vi "ScannerMain.vi"() -> ()   [LabVIEW 2012]
uses:
  Strict Type Def - Scan Parameters Cluster.ctl
  Strict Type Def - Optimize Parameters Cluster.ctl
  Rabi Window Parameters.ctl
  ESR Window Parameters.ctl
  Spin Echo Window Parameters.ctl
  Window Parameters-CPMG.ctl
  SaveContrastOptions.ctl
  Window Parameters-XY4.ctl
  ESR Processing Params.ctl
  ESR Processing State.ctl
  ESR Modified Window Parameters.ctl
  States.ctl
  Global Vars.vi
  Channels.vi
panel:
  in  "Program":T1(tab)
  in  "Z Voltage":dbl min=-10.0 max=10.0 step=0.1
  in  "Continuous":bool
  in  "Green Laser (low-T)":bool caption="Scan"
  in  "Microwave":bool caption="Scan"
  in  "Green Laser":bool caption="Scan"
  out "Counts Intensity Graph":i32[][](graph)
  in  "Scan Parameters":T2={"X Max"=1.0, "X Min"=-1.0, "X Step"=0.01, "Y Max"=1.5, "Y Min"=-1.5, "Y Step"=0.015, "Dwell Time (ms) "=1} {"Dwell Time (ms)" min=0; "Y Step" min=0.0; "X Step" min=0.0}
  in  "Optimize":bool
  in  "Scan":bool
  in  "Count":bool caption="Optimize"
  out "Counts Chart":u32(graph)=76190
  out "Counts/s":i32=76190
  in  "Optimize Parameters":T3={"Volt Step"={"X"=0.005, "Y"=0.005, "Z"=0.01}, "Num Iterations"=5, "Dwell Time (ms)"=25, "Volts Range"={"X"=0.05, "Y"=0.05, "Z"=0.0}, "Method"={"X"=enum."Max", "Y"=enum."Max", "Z"=enum."Max"}} {"Volts Range"."Z" min=0.0; "Volts Range"."Y" min=0.0; "Volts Range"."X" min=0.0; "Dwell Time (ms)" min=0; "Num Iterations" min=1 step=1; "Volt Step"."Z" min=1e-05; "Volt Step"."Y" min=1e-06; "Volt Step"."X" min=1e-06}
  in  "ESR Post-Processing Parameters":T4={"Cut-off Threshhold"=1.3, "Processing Type"=enum."Off"}
  in  "ESR":bool caption="Scan"
  in  "ESR spectrum spreadsheet":path=path "C:/Users/Loncar/Dropbox/Raw data/2014-09-25 Measurements on R5C2L9 beam 9 NV/ESR_r5c2l9_beam9_55uW_m12dBm_oldPCBonSichips_hires.txt"
  in  "Save ESR spectrum data":bool
  in  "ESR spectrum graph":path=path "C:/Users/Loncar/Dropbox/Raw data/2014-09-25 Measurements on R5C2L9 beam 9 NV/ESR_r5c2l9_beam9_55uW_m12dBm_oldPCBonSichips_hires.jpg"
  in  "Save ESR spectrum graph":bool
  out "Avg ESR spectrum":cluster{"Y":dbl[], "Y":dbl[]}[](graph)=[{"Y"=[2.86, 2.8602499999999997, 2.8605, 2.86075, 2.8609999999999998, 2.86125, 2.8615, 2.86175, 2.862, 2.86225, 2.8625, 2.8627499999999997, 2.863, 2.86325, 2.8634999999999997, 2.86375, 2.864, 2.8642499999999997, 2.8645, 2.86475, 2.8649999999999998, 2.86525, 2.8655, 2.86575, 2.8659999999999997, 2.86625, 2.8665, 2.8667499999999997, 2.867, 2.86725, 2.8674999999999997, 2.86775, 2.868, 2.8682499999999997, 2.8685, 2.86875, 2.8689999999999998, 2.86925, 2.8695, 2.86975, 2.87, 2.87025, 2.8705, 2.8707499999999997, 2.871, 2.87125, 2.8714999999999997, 2.87175, 2.872, 2.8722499999999997, 2.8725, 2.87275, 2.8729999999999998, 2.87325, 2.8735, 2.87375, 2.8739999999999997, 2.87425, 2.8745, 2.8747499999999997, 2.875, 2.87525, 2.8754999999999997, 2.87575, 2.876, 2.8762499999999998, 2.8765, 2.87675, 2.877, 2.87725, 2.8775, 2.87775, 2.878, 2.87825, 2.8785, 2.8787499999999997, 2.879, 2.87925, 2.8794999999999997, 2.87975, 2.88], "Y"=[171.2, 172.675, 175.59166666666667, 174.09166666666667, 175.0, 174.94166666666666, 175.05833333333334, 176.20833333333334, 174.75833333333333, 172.9, 173.675, 175.35, 174.325, 172.54166666666666, 173.83333333333334, 172.03333333333333, 173.89166666666668, 174.84166666666667, 173.04166666666666, 173.16666666666666, 171.03333333333333, 171.68333333333334, 169.74166666666667, 168.125, 167.25833333333333, 165.89166666666668, 163.9, 160.34166666666667, 155.55, 154.05, 152.5, 153.3, 153.525, 157.55833333333334, 161.56666666666666, 157.38333333333333, 157.175, 158.2, 154.24166666666667, 152.09166666666667, 147.9, 147.6, 147.875, 147.125, 149.8, 152.39166666666668, 156.35, 154.675, 157.55833333333334, 161.69166666666666, 160.13333333333333, 160.275, 160.2, 156.75833333333333, 156.76666666666668, 152.64166666666668, 149.14166666666668, 153.64166666666668, 155.76666666666668, 158.53333333333333, 162.56666666666666, 165.725, 168.45, 166.98333333333332, 168.93333333333334, 171.05833333333334, 172.13333333333333, 171.3, 172.825, 172.78333333333333, 171.06666666666666, 173.50833333333333, 171.28333333333333, 173.075, 172.475, 171.44166666666666, 173.40833333333333, 175.19166666666666, 172.86666666666667, 174.90833333333333, 174.175]}]
  out "Counts vs. frequency":i32[][](graph)
  in  "# freq points":i32=81
  in  "MW start freq (GHz)":dbl=2.86
  in  "MW stop freq (GHz)":dbl=2.88
  in  "# scans before track":i32=20
  in  "#scan iterations":i32=20
  in  "ESR Parameters":T6={"Window 1 time (s)"=0.012, "Window 2 time (s)"=5e-06, "Window 3 time (s) "=0.02, "Window 4 time (s)"=5e-07, "Window 4 channels"=[FALSE, FALSE, FALSE, TRUE], "Window 3 channels"=[FALSE, FALSE, TRUE, TRUE], "Window 2 channels"=[FALSE, FALSE, FALSE, TRUE], "Window 1 channels"=[FALSE, TRUE, FALSE, TRUE], "Path to ESR Burner"=path "C:/Users/Loncar/Desktop/ESR VIs - Srujan/Sam Kim/PB/ESRFreq.exe"}
  in  "ESR Save Data 2":T7={"Save avg spectrum graph"=FALSE, "Path for avg spectrum graph"=path "C:/experiment/data/may_15_2012/SIL1_NV1_pippin_uW_off", "Save data to spreadsheet"=FALSE, "Path for avg spectrum spreadsheet"=path "C:/experiment/data/may_15_2012/SIL1_NV1_pippin_uW_off"}
  out "Avg ESR spectrum 2-2":cluster{"Y":dbl[], "Y":dbl[]}[](graph)=[{"Y"=[2.86, 2.8602499999999997, 2.8605, 2.86075, 2.8609999999999998, 2.86125, 2.8615, 2.86175, 2.862, 2.86225, 2.8625, 2.8627499999999997, 2.863, 2.86325, 2.8634999999999997, 2.86375, 2.864, 2.8642499999999997, 2.8645, 2.86475, 2.8649999999999998, 2.86525, 2.8655, 2.86575, 2.8659999999999997, 2.86625, 2.8665, 2.8667499999999997, 2.867, 2.86725, 2.8674999999999997, 2.86775, 2.868, 2.8682499999999997, 2.8685, 2.86875, 2.8689999999999998, 2.86925, 2.8695, 2.86975, 2.87, 2.87025, 2.8705, 2.8707499999999997, 2.871, 2.87125, 2.8714999999999997, 2.87175, 2.872, 2.8722499999999997, 2.8725, 2.87275, 2.8729999999999998, 2.87325, 2.8735, 2.87375, 2.8739999999999997, 2.87425, 2.8745, 2.8747499999999997, 2.875, 2.87525, 2.8754999999999997, 2.87575, 2.876, 2.8762499999999998, 2.8765, 2.87675, 2.877, 2.87725, 2.8775, 2.87775, 2.878, 2.87825, 2.8785, 2.8787499999999997, 2.879, 2.87925, 2.8794999999999997, 2.87975, 2.88], "Y"=[171.2, 172.675, 175.59166666666667, 174.09166666666667, 175.0, 174.94166666666666, 175.05833333333334, 176.20833333333334, 174.75833333333333, 172.9, 173.675, 175.35, 174.325, 172.54166666666666, 173.83333333333334, 172.03333333333333, 173.89166666666668, 174.84166666666667, 173.04166666666666, 173.16666666666666, 171.03333333333333, 171.68333333333334, 169.74166666666667, 168.125, 167.25833333333333, 165.89166666666668, 163.9, 160.34166666666667, 155.55, 154.05, 152.5, 153.3, 153.525, 157.55833333333334, 161.56666666666666, 157.38333333333333, 157.175, 158.2, 154.24166666666667, 152.09166666666667, 147.9, 147.6, 147.875, 147.125, 149.8, 152.39166666666668, 156.35, 154.675, 157.55833333333334, 161.69166666666666, 160.13333333333333, 160.275, 160.2, 156.75833333333333, 156.76666666666668, 152.64166666666668, 149.14166666666668, 153.64166666666668, 155.76666666666668, 158.53333333333333, 162.56666666666666, 165.725, 168.45, 166.98333333333332, 168.93333333333334, 171.05833333333334, 172.13333333333333, 171.3, 172.825, 172.78333333333333, 171.06666666666666, 173.50833333333333, 171.28333333333333, 173.075, 172.475, 171.44166666666666, 173.40833333333333, 175.19166666666666, 172.86666666666667, 174.90833333333333, 174.175]}] caption="Avg ESR spectrum 2"
  out "Counts vs. frequency 2-2":i32[][](graph) caption="Counts vs. frequency 2"
  in  "ESR Save Data 1":T7={"Save avg spectrum graph"=FALSE, "Path for avg spectrum graph"=path "C:/experiment/data/may_15_2012/SIL1_NV1_pippin_uW_off", "Save data to spreadsheet"=FALSE, "Path for avg spectrum spreadsheet"=path "C:/experiment/data/may_15_2012/SIL1_NV1_pippin_uW_off"}
  in  "ESR Post-Processing Parameters 2":T4={"Cut-off Threshhold"=1.3, "Processing Type"=enum."Off"}
  in  "ESR 2":bool caption="Scan"
  out "Avg ESR spectrum 2-1":cluster{"Y":dbl[], "Y":dbl[]}[](graph)=[{"Y"=[2.86, 2.8602499999999997, 2.8605, 2.86075, 2.8609999999999998, 2.86125, 2.8615, 2.86175, 2.862, 2.86225, 2.8625, 2.8627499999999997, 2.863, 2.86325, 2.8634999999999997, 2.86375, 2.864, 2.8642499999999997, 2.8645, 2.86475, 2.8649999999999998, 2.86525, 2.8655, 2.86575, 2.8659999999999997, 2.86625, 2.8665, 2.8667499999999997, 2.867, 2.86725, 2.8674999999999997, 2.86775, 2.868, 2.8682499999999997, 2.8685, 2.86875, 2.8689999999999998, 2.86925, 2.8695, 2.86975, 2.87, 2.87025, 2.8705, 2.8707499999999997, 2.871, 2.87125, 2.8714999999999997, 2.87175, 2.872, 2.8722499999999997, 2.8725, 2.87275, 2.8729999999999998, 2.87325, 2.8735, 2.87375, 2.8739999999999997, 2.87425, 2.8745, 2.8747499999999997, 2.875, 2.87525, 2.8754999999999997, 2.87575, 2.876, 2.8762499999999998, 2.8765, 2.87675, 2.877, 2.87725, 2.8775, 2.87775, 2.878, 2.87825, 2.8785, 2.8787499999999997, 2.879, 2.87925, 2.8794999999999997, 2.87975, 2.88], "Y"=[171.2, 172.675, 175.59166666666667, 174.09166666666667, 175.0, 174.94166666666666, 175.05833333333334, 176.20833333333334, 174.75833333333333, 172.9, 173.675, 175.35, 174.325, 172.54166666666666, 173.83333333333334, 172.03333333333333, 173.89166666666668, 174.84166666666667, 173.04166666666666, 173.16666666666666, 171.03333333333333, 171.68333333333334, 169.74166666666667, 168.125, 167.25833333333333, 165.89166666666668, 163.9, 160.34166666666667, 155.55, 154.05, 152.5, 153.3, 153.525, 157.55833333333334, 161.56666666666666, 157.38333333333333, 157.175, 158.2, 154.24166666666667, 152.09166666666667, 147.9, 147.6, 147.875, 147.125, 149.8, 152.39166666666668, 156.35, 154.675, 157.55833333333334, 161.69166666666666, 160.13333333333333, 160.275, 160.2, 156.75833333333333, 156.76666666666668, 152.64166666666668, 149.14166666666668, 153.64166666666668, 155.76666666666668, 158.53333333333333, 162.56666666666666, 165.725, 168.45, 166.98333333333332, 168.93333333333334, 171.05833333333334, 172.13333333333333, 171.3, 172.825, 172.78333333333333, 171.06666666666666, 173.50833333333333, 171.28333333333333, 173.075, 172.475, 171.44166666666666, 173.40833333333333, 175.19166666666666, 172.86666666666667, 174.90833333333333, 174.175]}] caption="Avg ESR spectrum 1"
  out "Counts vs. frequency 2-1":i32[][](graph) caption="Counts vs. frequency 1"
  in  "# freq points 2":i32=81 caption="# freq points"
  in  "MW start freq (GHz) 2":dbl=2.86 caption="MW start freq (GHz)"
  in  "MW stop freq (GHz) 2":dbl=2.88 caption="MW stop freq (GHz)"
  in  "# scans before track 2":i32=20
  in  "#scan iterations 2":i32=20 caption="#scan iterations"
  in  "ESR Modified Parameters":T8={"Window 1 time (s)"=0.012, "Window 2 time (s)"=5e-06, "Window 3 time (s) "=0.02, "Window 4 time (s)"=5e-07, "Window 4 channels"=[FALSE, FALSE, FALSE, TRUE], "Window 3 channels"=[FALSE, FALSE, TRUE, TRUE], "Window 2 channels"=[FALSE, FALSE, FALSE, TRUE], "Window 1 channels"=[FALSE, TRUE, FALSE, TRUE], "Path to ESR Burner"=path "C:/Users/Loncar/Desktop/ESR VIs - Srujan/Sam Kim/PB/ESR_modified_burn.exe", "Window 5 time (s)"=1.0, "Drive channel"=4} {"Drive channel" max=8}
  out "Rabi # scans done":u32=4
  in  "Save Rabi Contrast Options":T9={"Save contrast graph"=FALSE, "Path for contrast graph"=path "C:/Users/Loncar/Dropbox/Raw data/2014-09-25 Measurements on R5C2L9 beam 9 NV/Rabi_r5c2l9_beam9_100uW_3dBm2p87050GHz_oldPCBonSichips.jpg", "Save contrast data"=FALSE, "Path for contrast data"=path "C:/Users/Loncar/Dropbox/Raw data/2014-09-25 Measurements on R5C2L9 beam 9 NV/Rabi_r5c2l9_beam9_100uW_3dBm2p87050GHz_oldPCBonSichips.txt"}
  in  "# scan iterations":i32=100
  in  "Rabi Parameters":T10={"Window 1 time (s)"=3e-06, "Window 2 time (s)"=1e-06, "Window 3 min time (s) "=1.2e-08, "Window 3 max time (s)"=2e-07, "Window 4 time (s)"=7.5e-07, "Window 5 time (s)"=2e-07, "Window 6 time (s)"=3e-06, "Window 7 time (s)"=2e-07, "Window 8 time (s)"=1e-07, "# samples before track"=100000, "# time axis points"=94, "Window 1 active channels"=[TRUE, FALSE, FALSE, TRUE], "Window 2 active channels"=[TRUE], "Window 3 active channels"=[FALSE], "Window 4 active channels"=[TRUE, FALSE, FALSE, TRUE], "Window 5 active channels "=[TRUE, FALSE, TRUE, TRUE], "Window 6 active channels"=[TRUE, FALSE, FALSE, TRUE], "Window 7 active channels"=[TRUE, FALSE, TRUE, TRUE], "Window 8 active channels"=[TRUE], "Path to Rabi Burner"=path "C:/Users/Loncar/Desktop/ESR VIs - Srujan/Sam Kim/PB/RabiBurn.exe"}
  out "Rabi Normalized contrast":cluster{"Y":dbl[], "Y":dbl[]}[](graph)=[{"Y"=[0.012, 0.014021505376344086, 0.016043010752688172, 0.018064516129032256, 0.020086021505376344, 0.02210752688172043, 0.024129032258064516, 0.0261505376344086, 0.028172043010752684, 0.030193548387096772, 0.03221505376344086, 0.03423655913978495, 0.03625806451612903, 0.038279569892473116, 0.0403010752688172, 0.04232258064516129, 0.04434408602150538, 0.04636559139784946, 0.04838709677419355, 0.050408602150537635, 0.05243010752688172, 0.05445161290322581, 0.05647311827956989, 0.05849462365591398, 0.06051612903225806, 0.06253763440860215, 0.06455913978494623, 0.06658064516129032, 0.0686021505376344, 0.0706236559139785, 0.07264516129032259, 0.07466666666666666, 0.07668817204301075, 0.07870967741935485, 0.08073118279569892, 0.08275268817204301, 0.0847741935483871, 0.08679569892473118, 0.08881720430107527, 0.09083870967741935, 0.09286021505376345, 0.09488172043010752, 0.09690322580645161, 0.0989247311827957, 0.10094623655913978, 0.10296774193548387, 0.10498924731182795, 0.10701075268817205, 0.10903225806451612, 0.11105376344086021, 0.1130752688172043, 0.11509677419354838, 0.11711827956989247, 0.11913978494623655, 0.12116129032258065, 0.12318279569892474, 0.1252043010752688, 0.12722580645161288, 0.12924731182795698, 0.13126881720430106, 0.13329032258064516, 0.13531182795698926, 0.1373333333333333, 0.1393548387096774, 0.1413763440860215, 0.14339784946236558, 0.14541935483870969, 0.14744086021505376, 0.14946236559139783, 0.15148387096774193, 0.15350537634408604, 0.1555268817204301, 0.15754838709677418, 0.15956989247311826, 0.16159139784946236, 0.16361290322580646, 0.16563440860215053, 0.1676559139784946, 0.1696774193548387, 0.17169892473118278, 0.17372043010752689, 0.175741935483871, 0.17776344086021503, 0.17978494623655913, 0.1818064516129032, 0.1838279569892473, 0.1858494623655914, 0.18787096774193546, 0.18989247311827956, 0.19191397849462366, 0.19393548387096773, 0.19595698924731184, 0.1979784946236559, 0.19999999999999998], "Y"=[-0.08553971486761709, 0.011664899257688167, 0.13925438596491221, 0.06770255271920085, 0.08048511576626233, -0.04601226993865021, 0.030916844349680114, -0.032734952481520585, 0.02651933701657463, 0.013978494623655904, -0.07476635514018694, 0.012074643249176665, 0.015856236786469385, -0.016685205784204595, -0.03520352035203522, -0.0965447154471545, -0.10626992561105213, -0.11300639658848623, -0.09570957095709565, -0.12087912087912084, -0.17196056955093092, -0.12861736334405144, -0.1610169491525424, -0.12705366922234393, -0.10515463917525783, -0.1439312567132116, -0.09857612267250825, -0.08786127167630059, -0.14553472987872113, -0.1956521739130434, -0.19296375266524526, -0.23037716615698273, -0.23809523809523814, -0.2172489082969433, -0.25467775467775466, -0.22137404580152667, -0.30620985010706636, -0.23583934088568478, -0.30512016718913265, -0.31137088204038255, -0.2988260405549626, -0.21221864951768493, -0.2749731471535982, -0.29181084198385243, -0.31327800829875513, -0.3020719738276989, -0.20136518771331055, -0.38453713123092575, -0.3240641711229947, -0.3050483351235231, -0.41277890466531436, -0.37362637362637363, -0.3563096500530223, -0.3563714902807775, -0.3038793103448276, -0.3427922814982974, -0.39764201500535906, -0.3432203389830508, -0.37060702875399354, -0.2960893854748603, -0.3371017471736897, -0.3094462540716613, -0.3705636743215031, -0.37731958762886597, -0.3152866242038217, -0.2636871508379888, -0.35586481113320073, -0.29205366357069146, -0.34840698869475845, -0.35966735966735963, -0.36185567010309283, -0.2676537585421412, -0.3159541188738269, -0.30687830687830686, -0.3009605122732124, -0.29538131041890436, -0.24860646599777034, -0.2631578947368421, -0.26400862068965514, -0.3076923076923076, -0.208955223880597, -0.2309322033898305, -0.29610115911485774, -0.23751274209989817, -0.20000000000000007, -0.18343815513626838, -0.23179487179487177, -0.2694248234106962, -0.1670258620689655, -0.2071503680336488, -0.20141700404858295, -0.17057569296375263, -0.1054384017758047, -0.15129533678756485]}]
  in  "Rabi":bool caption="Scan"
  in  "Rabi Pause":bool
  out "Rabi Last counts/s":u32 caption="Last counts/s"
  out "Last counts/s":u32
  out "SpinEcho scans done":u32=104
  in  "Pause Spin Echo":bool
  in  "SpinEcho Save Options":T9={"Save contrast graph"=FALSE, "Path for contrast graph"=path "C:/Users/Loncar/Dropbox/Raw data/2014-09-25 Measurements on R5C2L9 beam 9 NV/SpinEcho_r5c2l9_beam9_100uW_3dBm2p87050GHz_oldPCBonSichips_10us.jpg", "Save contrast data"=FALSE, "Path for contrast data"=path "C:/Users/Loncar/Dropbox/Raw data/2014-09-25 Measurements on R5C2L9 beam 9 NV/SpinEcho_r5c2l9_beam9_100uW_3dBm2p87050GHz_oldPCBonSichips_10us.txt"}
  in  "# SpinEcho scan iterations":i32=200
  in  "Spin Echo Parameters":T11={"Path to Spin Echo Burner"=path "C:/Users/Loncar/Desktop/ESR VIs - Srujan/Sam Kim/PB/SpinEchoBurn.exe", "Window 1 time (s)"=3e-06, "Window 1 active channels"=[TRUE, FALSE, FALSE, TRUE], "Window 10 time (s)"=3e-06, "Window 10 active channels"=[TRUE, FALSE, FALSE, TRUE], "# samples"=50000, "Window 2 time (s)"=1e-06, "Window 2 active channels"=[TRUE], "Window 4 min time (s) "=1.2e-08, "Window 4 active channels"=[TRUE], "Window 8 time (s)"=7.5e-07, "Window 8 active channels"=[TRUE, FALSE, FALSE, TRUE], "Window 9 time (s)"=2e-07, "Window 9 active channels "=[TRUE, FALSE, TRUE, TRUE], "# time axis points"=300, "Window 11 time (s)"=2e-07, "Window 11 active channels"=[TRUE, FALSE, TRUE, TRUE], "Window 12 time (s)"=1e-07, "Window 12 active channels"=[TRUE], "Window 4 max time (s)"=1e-05, "Window 3 time (s)"=6.5e-08, "Window 5 time (s)"=2.6e-07, "Window 3 active channels"=[FALSE, FALSE, FALSE, FALSE], "Window 5 active channels"=[FALSE, FALSE, FALSE, FALSE], "Window 7 time (s)"=6.5e-08, "Window 7 active channels"=[FALSE, FALSE, FALSE, FALSE]}
  out "Spin Echo contrast":cluster{"Y":dbl[], "Y":dbl[]}[](graph)
  in  "Spin Echo":bool caption="Scan"
  out "CPMG scans done":u32=88
  in  "Save CPMG Contrast Options":T9={"Save contrast graph"=FALSE, "Path for contrast graph"=path "C:/Users/Public/Documents/Srujan/2014-06-22/NV3_CPMG_n2_2p83GHz3dBm_pi64ns_100us.jpg", "Save contrast data"=FALSE, "Path for contrast data"=path "C:/Users/Public/Documents/Srujan/2014-06-22/NV3_CPMG_n2_2p83GHz3dBm_pi64ns_100us.txt"}
  out "CPMG contrast":cluster{"Y":dbl[], "Y":dbl[]}[](graph)
  in  "CPMG":bool caption="Scan"
  in  "# scan iterations":i32=200
  in  "CPMG Parameters":T12={"Path to CPMG Burner"=path "C:/Users/Loncar/Desktop/ESR VIs - Srujan/Sam Kim/PB/SpinEchoBurn.exe", "Window 1 time (s)"=3e-06, "Window 1 active channels"=[FALSE, FALSE, FALSE, TRUE], "Window 10 time (s)"=3e-06, "Window 10 active channels"=[FALSE, FALSE, FALSE, TRUE], "Window 2 time (s)"=1e-06, "Window 2 active channels"=[], "Window 4 min time (s) "=1.2e-08, "Window 4 active channels"=[FALSE], "Window 8 time (s)"=7.5e-07, "Window 8 active channels"=[FALSE, FALSE, FALSE, TRUE], "Window 9 time (s)"=3e-07, "Window 9 active channels "=[FALSE, FALSE, TRUE, TRUE], "# delay time points"=100, "Window 11 time (s)"=3e-07, "Window 11 active channels"=[FALSE, FALSE, TRUE, TRUE], "Window 12 time (s)"=1e-07, "Window 12 active channels"=[], "Window 4 max time (s)"=0.0001, "Window 3 time (s)"=3.2e-08, "Window 5 time (s)"=6.4e-08, "Window 3 active channels"=[TRUE, FALSE, FALSE, FALSE], "Window 5 active channels"=[TRUE, FALSE, FALSE, FALSE], "# pi pulses"=2, "# samples before track"=20000} {"# pi pulses" min=1; "# delay time points" min=2}
  in  "Save XY-4 Contrast Options":T9={"Save contrast graph"=FALSE, "Path for contrast graph"=path "C:/experiment/data/may_15_2012/SIL1_NV1_pippin_uW_off", "Save contrast data"=FALSE, "Path for contrast data"=path "C:/experiment/data/may_15_2012/SIL1_NV1_pippin_uW_off"}
  out "XY-4 Normalized contrast":cluster{"Y":dbl[], "Y":dbl[]}[](graph)
  in  "XY-4":bool caption="Scan"
  in  "# scan iterations":i32
  in  "XY-4 Parameters":T13={"Path to CPMG Burner"=path "C:/Users/Loncar/Desktop/ESR VIs - Srujan/Sam Kim/PB/SpinEchoBurn.exe", "Window 1 time (s)"=3e-06, "Window 1 active channels"=[FALSE, FALSE, FALSE, TRUE], "Window 10 time (s)"=3e-06, "Window 10 active channels"=[FALSE, FALSE, FALSE, TRUE], "Window 2 time (s)"=0.0, "Window 2 active channels"=[], "Window 4 min time (s) "=0.0, "Window 4 active channels"=[FALSE], "Window 8 time (s)"=7.5e-07, "Window 8 active channels"=[FALSE, FALSE, FALSE, TRUE], "Window 9 time (s)"=2e-07, "Window 9 active channels "=[FALSE, FALSE, TRUE, TRUE], "# time points"=2, "Window 11 time (s)"=0.0, "Window 11 active channels"=[FALSE, FALSE, TRUE, TRUE], "Window 12 time (s)"=1e-07, "Window 12 active channels"=[], "Window 4 max time (s)"=0.0, "Window 3 time (s)"=0.0, "Window 5 time (s)"=5e-06, "Window 3 active channels"=[TRUE, FALSE, FALSE, FALSE], "Window 5c active channels"=[TRUE, FALSE, FALSE, FALSE], "# pulse sequences"=1, "# samples before track"=0, "Window 5a active channels"=[TRUE, FALSE, FALSE, FALSE]} {"# pulse sequences" min=1; "# time points" min=2}
  in  "Z AO Channel":tag="Dev1/ao2"
  in  "Laser voltage":tag="Dev1/ao2"
  in  "Counter(s)":tag="Dev1/ctr0"
  in  "X AO Channel":tag="Dev1/ao0"
  in  "Y AO Channel":tag="Dev1/ao1"
  in  "Sample clock line":tag="/Dev1/PFI9"
  in  "spinapi.dll":path=path "C:/SpinCore/SpinAPI/dll/spinapi64.dll"
  in  "HoldChannel.exe":path=path "C:/Users/Loncar/Desktop/ESR VIs - Srujan/Sam Kim/PB/HoldChannel.exe"
  # "Note for Z: 1 V = 10 um"
  # "X, Y, and Z display values\nonly update after manual\noptimization"
  # "Default PB connections:\nPB0 - MW switch\nPB3 - Green AOM\n\nDefault for low-T:\nPB1 - Green AOM"
  # "ESR spectrum measurement"
  # "Default PB connections:\nPB0 - MW switch\nPB1 - MW freq step\nPB2 - Counter sample clk\nPB3 - Green AOM"
  # "Pulse sequence parameters - Window durations and PB channel states"
  # "Green AOM, MW switch are always on!"
  # "(to spreadsheet)"
  # "Remove Outlier Scan: If there are outlier data\n    in a scan, then removes that scan\nRemove Outlier Data: If there are outlier data,\n    then replaces the data with the mean of\n    that scan"
  # "* <data>"
  # "MW freq step\ndwell time"
  # "MW freq step"
  # "Wait"
  # "Fluorescence\ncounting"
  # "Ctr sample clk"
  # "Wait"
  # "ESR 2 (modified) measurement"
  # "Default PB connections:\nPB0 - MW switch\nPB1 - MW freq step\nPB2 - Counter sample clk\nPB3 - Green AOM\nPB4 - Piezo drive"
  # "Modified version: Alternates frequency sweep with channel on/off for driving cantilever"
  # "Pulse sequence parameters - Window durations and PB channel states"
  # "Green AOM, MW switch are always on!"
  # "Remove Outlier Scan: If there are outlier data\n    in a scan, then removes that scan\nRemove Outlier Data: If there are outlier data,\n    then replaces the data with the mean of\n    that scan"
  # "* <data>"
  # "MW freq step\ndwell time"
  # "MW freq step"
  # "Wait"
  # "Fluorescence\ncounting"
  # "Ctr sample clk"
  # "Wait"
  # "Wait between\nfreq sweeps"
  # "On/off between freq sweeps (off first)"
  # "Rabi measurement"
  # "Default PB connections:\nPB0 - MW switch\nPB1 - unused\nPB2 - Counter sample clk\nPB3 - Green AOM"
  # "to spreadsheet"
  # "Initialization"
  # "Green AOM"
  # "Wait"
  # "All off"
  # "MW pulsing"
  # "MW"
  # "Wait"
  # "Green AOM"
  # "Green AOM,\ncounter clk"
  # "Readout"
  # "Repump"
  # "Green AOM"
  # "Green AOM,\ncounter clk"
  # "Reference"
  # "All off"
  # "Wait (nominal)"
  # "Spin Echo measurement"
  # "Default PB connections:\nPB0 - MW switch\nPB1 - unused\nPB2 - Counter sample clk\nPB3 - Green AOM"
  # "to spreadsheet"
  # "Green AOM"
  # "Initialization"
  # "All off"
  # "Wait"
  # "MW"
  # "MW pulse 1"
  # "All off"
  # "Free precession 1"
  # "max: ~350"
  # "MW pulse 2"
  # "MW"
  # "Free precession 2: Window 6"
  # "MW"
  # "MW pulse 1"
  # "Green AOM"
  # "Wait"
  # "Green AOM,\ncounter clk"
  # "Readout"
  # "Green AOM"
  # "Repump"
  # "Green AOM,\ncounter clk"
  # "Reference"
  # "Wait (nominal)"
  # "All off"
  # "CPMG measurement"
  # "Default PB connections:\nPB0 - MW switch\nPB1 - MW 90deg phase shifted\nPB2 - Counter sample clk\nPB3 - Green AOM"
  # "to spreadsheet"
  # "Green AOM"
  # "Initialization"
  # "All off"
  # "Wait"
  # "MW pulse 1\n(pi/2)"
  # "MW"
  # "Free precession\n(Tau/2)"
  # "All off"
  # "max: ~350"
  # "MW pulse 2\n(pi90)"
  # "MW90"
  # "Free precession (Tau/2)\nMW pulse 1 (pi/2)"
  # "Window 6 = Window 4\nWindow 7 = Window 3"
  # "All off\nMW"
  # "Green AOM"
  # "Wait for green"
  # "Green AOM,\ncounter clk"
  # "Readout"
  # "Green AOM"
  # "Repump"
  # "Green AOM,\ncounter clk"
  # "Reference"
  # "Wait (nominal)"
  # "All off"
  # "XY-4 measurement"
  # "Default PB connections:\nPB0 - MW switch\nPB1 - MW 90deg phase shifted\nPB2 - Counter sample clk\nPB3 - Green AOM"
  # "to spreadsheet"
  # "pulse=XYXY"
  # "max: ~350"
  # "x 4=#pi pulses"
  # "Green AOM"
  # "Initialization"
  # "All off"
  # "Wait"
  # "MW pulse 1\n(pi/2)"
  # "MW"
  # "Free precession\n(T/2)"
  # "All off"
  # "MW (X)"
  # "MW pulse 2\n(pi)"
  # "MW90 (Y)"
  # "Pulse Sequence=[T/2-Pi-T-Pi90-T-Pi-T-Pi90-T/2]^N\nMW pulse 1 (pi/2)"
  # "Window 4-5a-g-6\nWindow 7"
  # "Green AOM"
  # "Wait for green"
  # "Green AOM,\ncounter sample clk"
  # "Readout"
  # "Green AOM"
  # "Repump"
  # "Green AOM,\ncounter sample clk"
  # "Reference"
  # "Wait (nominal)"
  # "All off"
  # "TODO:\nHigh priority:\n(done) Show counts during pulsed experiments\nFigure out off-by-1 error in raster scan(?)\nImplement scanning with second arm\n\nMedium priority:\nChanges in Srujan's low-T experiments\n\nLow priority:\nContinuous Scan does not save image\nSave Counts Intensity Graph as image to clipbard\nAllow ESR+pulsed experiments to stop and save\n    (1. Stop at end of run; 2. Force stop)\nImplement new tracking algorithm for noisy data\n    (Ensemble NV centers)\nAllow stopping in middle of optimize\nAllow count concurrently with optimize/scan(?)"
  # "Author: Samuel Kim\nESR, Rabi, and Spin Echo experiments adapted from Srujan"
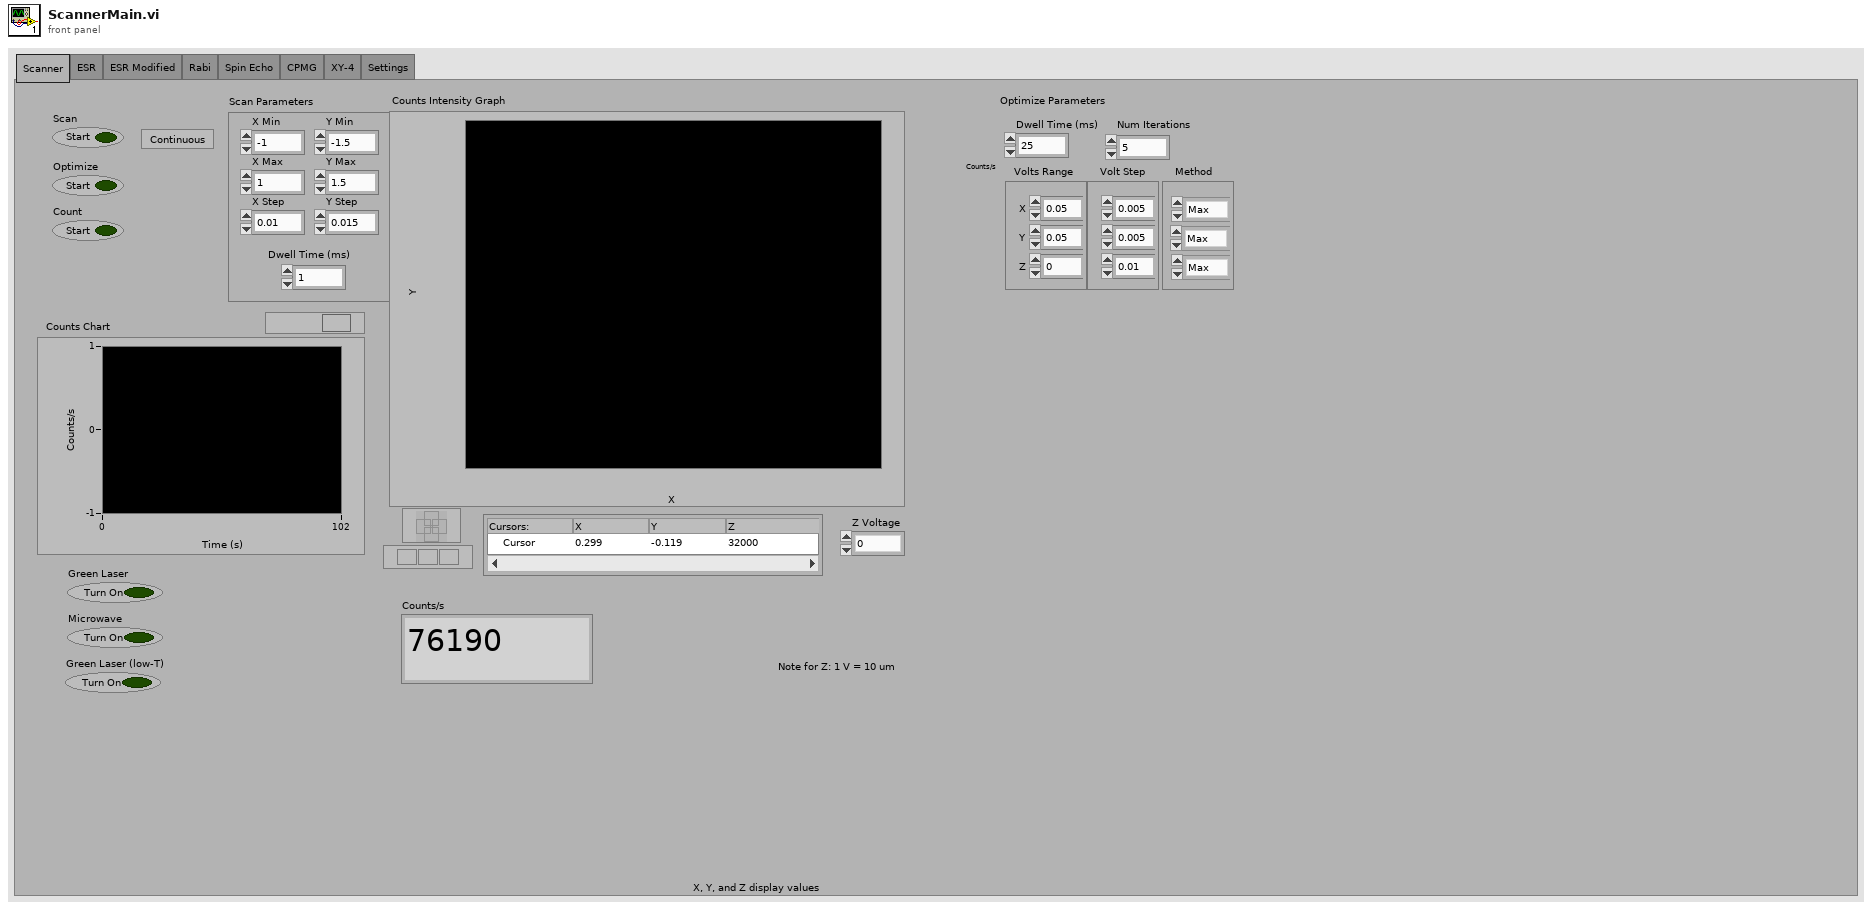
[diagram p1: front panel]
types:
  T1 = enum32{"Scanner", "ESR", "ESR Modified", "Rabi", "Spin Echo", "CPMG", "XY-4", "Settings"}
  T2 = typedef "Strict Type Def - Scan Parameters Cluster.ctl" = cluster{"X Max":dbl, "X Min":dbl, "X Step":dbl, "Y Max":dbl, "Y Min":dbl, "Y Step":dbl, "Dwell Time (ms) ":i32}
  T3 = typedef "Strict Type Def - Optimize Parameters Cluster.ctl" = cluster{"Volt Step":cluster{"X":dbl, "Y":dbl, "Z":dbl}, "Num Iterations":i32, "Dwell Time (ms)":i32, "Volts Range":cluster{"X":dbl, "Y":dbl, "Z":dbl}, "Method":cluster{"X":enum16{"Max", "Gaussian"}, "Y":enum16{"Max", "Gaussian"}, "Z":enum16{"Max", "Gaussian"}}}
  T4 = typedef "ESR Processing Params.ctl" = cluster{"Cut-off Threshhold":dbl, "Processing Type":T5}
  T5 = typedef "ESR Processing State.ctl" = enum16{"Off", "Remove Outlier Scan", "Remove Outlier Data"}
  T6 = typedef "ESR Window Parameters.ctl" = cluster{"Window 1 time (s)":dbl, "Window 2 time (s)":dbl, "Window 3 time (s) ":dbl, "Window 4 time (s)":dbl, "Window 4 channels":bool[], "Window 3 channels":bool[], "Window 2 channels":bool[], "Window 1 channels":bool[], "Path to ESR Burner":path}
  T7 = cluster{"Save avg spectrum graph":bool, "Path for avg spectrum graph":path, "Save data to spreadsheet":bool, "Path for avg spectrum spreadsheet":path}
  T8 = typedef "ESR Modified Window Parameters.ctl" = cluster{"Window 1 time (s)":dbl, "Window 2 time (s)":dbl, "Window 3 time (s) ":dbl, "Window 4 time (s)":dbl, "Window 4 channels":bool[], "Window 3 channels":bool[], "Window 2 channels":bool[], "Window 1 channels":bool[], "Path to ESR Burner":path, "Window 5 time (s)":dbl, "Drive channel":u8}
  T9 = typedef "SaveContrastOptions.ctl" = cluster{"Save contrast graph":bool, "Path for contrast graph":path, "Save contrast data":bool, "Path for contrast data":path}
  T10 = typedef "Rabi Window Parameters.ctl" = cluster{"Window 1 time (s)":dbl, "Window 2 time (s)":dbl, "Window 3 min time (s) ":dbl, "Window 3 max time (s)":dbl, "Window 4 time (s)":dbl, "Window 5 time (s)":dbl, "Window 6 time (s)":dbl, "Window 7 time (s)":dbl, "Window 8 time (s)":dbl, "# samples before track":i32, "# time axis points":i32, "Window 1 active channels":bool[], "Window 2 active channels":bool[], "Window 3 active channels":bool[], "Window 4 active channels":bool[], "Window 5 active channels ":bool[], "Window 6 active channels":bool[], "Window 7 active channels":bool[], "Window 8 active channels":bool[], "Path to Rabi Burner":path}
  T11 = typedef "Spin Echo Window Parameters.ctl" = cluster{"Path to Spin Echo Burner":path, "Window 1 time (s)":dbl, "Window 1 active channels":bool[], "Window 10 time (s)":dbl, "Window 10 active channels":bool[], "# samples":i32, "Window 2 time (s)":dbl, "Window 2 active channels":bool[], "Window 4 min time (s) ":dbl, "Window 4 active channels":bool[], "Window 8 time (s)":dbl, "Window 8 active channels":bool[], "Window 9 time (s)":dbl, "Window 9 active channels ":bool[], "# time axis points":i32, "Window 11 time (s)":dbl, "Window 11 active channels":bool[], "Window 12 time (s)":dbl, "Window 12 active channels":bool[], "Window 4 max time (s)":dbl, "Window 3 time (s)":dbl, "Window 5 time (s)":dbl, "Window 3 active channels":bool[], "Window 5 active channels":bool[], "Window 7 time (s)":dbl, "Window 7 active channels":bool[]}
  T12 = typedef "Window Parameters-CPMG.ctl" = cluster{"Path to CPMG Burner":path, "Window 1 time (s)":dbl, "Window 1 active channels":bool[], "Window 10 time (s)":dbl, "Window 10 active channels":bool[], "Window 2 time (s)":dbl, "Window 2 active channels":bool[], "Window 4 min time (s) ":dbl, "Window 4 active channels":bool[], "Window 8 time (s)":dbl, "Window 8 active channels":bool[], "Window 9 time (s)":dbl, "Window 9 active channels ":bool[], "# delay time points":i32, "Window 11 time (s)":dbl, "Window 11 active channels":bool[], "Window 12 time (s)":dbl, "Window 12 active channels":bool[], "Window 4 max time (s)":dbl, "Window 3 time (s)":dbl, "Window 5 time (s)":dbl, "Window 3 active channels":bool[], "Window 5 active channels":bool[], "# pi pulses":i32, "# samples before track":i32}
  T13 = typedef "Window Parameters-XY4.ctl" = cluster{"Path to CPMG Burner":path, "Window 1 time (s)":dbl, "Window 1 active channels":bool[], "Window 10 time (s)":dbl, "Window 10 active channels":bool[], "Window 2 time (s)":dbl, "Window 2 active channels":bool[], "Window 4 min time (s) ":dbl, "Window 4 active channels":bool[], "Window 8 time (s)":dbl, "Window 8 active channels":bool[], "Window 9 time (s)":dbl, "Window 9 active channels ":bool[], "# time points":i32, "Window 11 time (s)":dbl, "Window 11 active channels":bool[], "Window 12 time (s)":dbl, "Window 12 active channels":bool[], "Window 4 max time (s)":dbl, "Window 3 time (s)":dbl, "Window 5 time (s)":dbl, "Window 3 active channels":bool[], "Window 5c active channels":bool[], "# pulse sequences":i32, "# samples before track":i32, "Window 5a active channels":bool[]}
  T14 = typedef "States.ctl" = enum16{"Initialize", "Scan", "Count", "Optimize", "Hold", "ESR", "ESR 2", "Rabi", "Spin Echo", "Spectrum", "Stability", "CPMG", "XY-4", "Exit"}
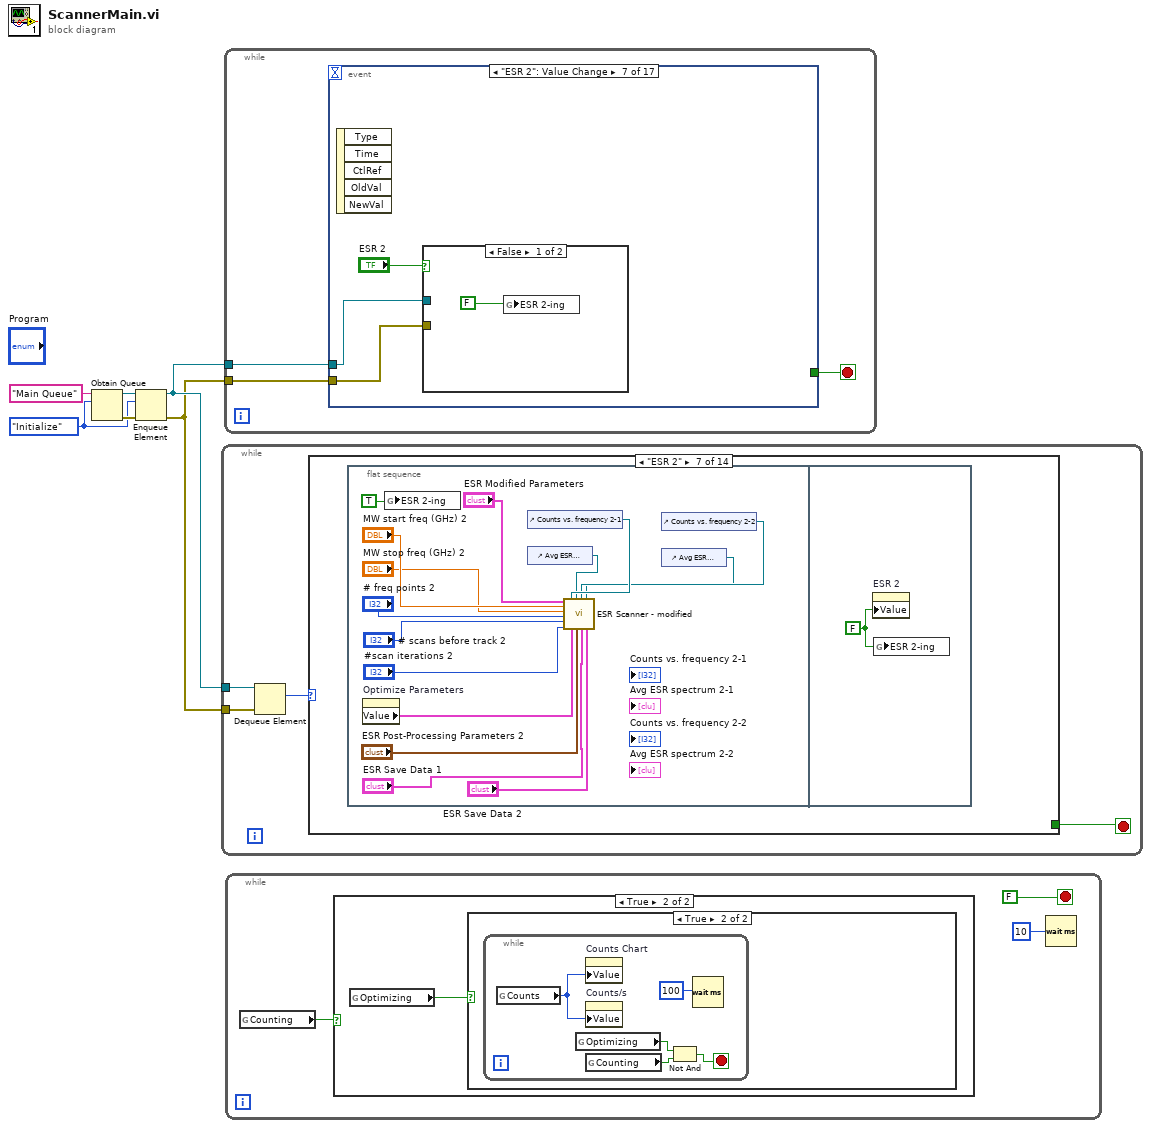
[diagram p0: block diagram]
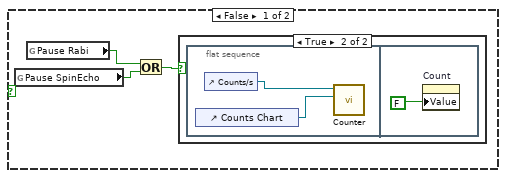
[diagram p3: hidden frame]
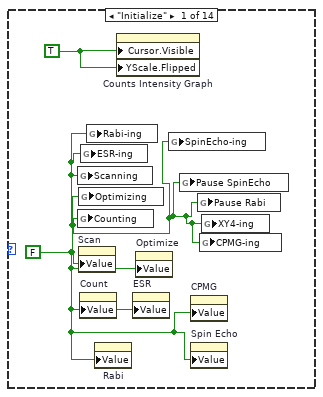
[diagram p5: hidden frame]
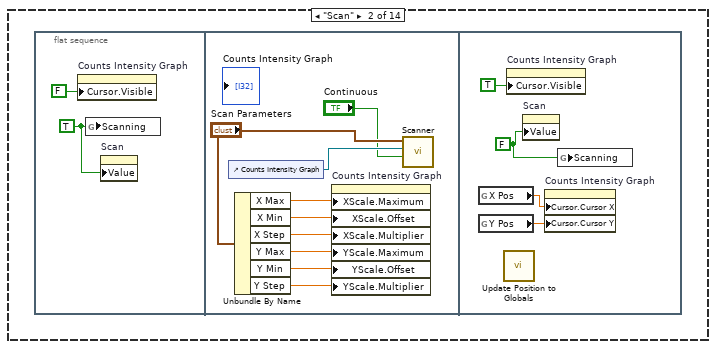
[diagram p6: hidden frame]
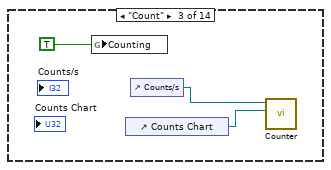
[diagram p7: hidden frame]
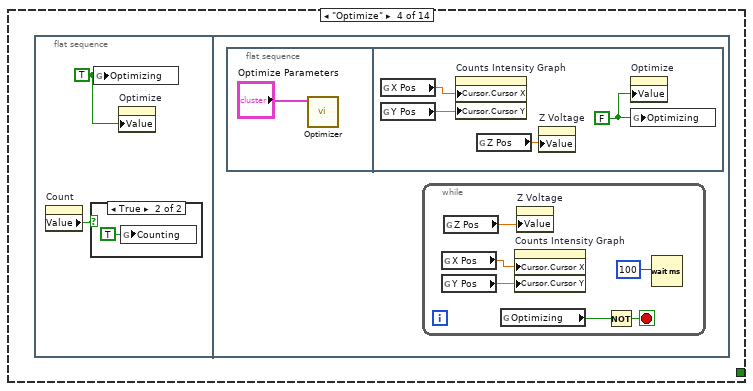
[diagram p8: hidden frame]
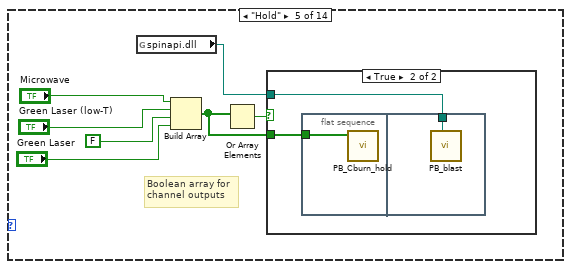
[diagram p10: hidden frame]
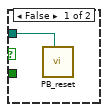
[diagram p11: hidden frame]
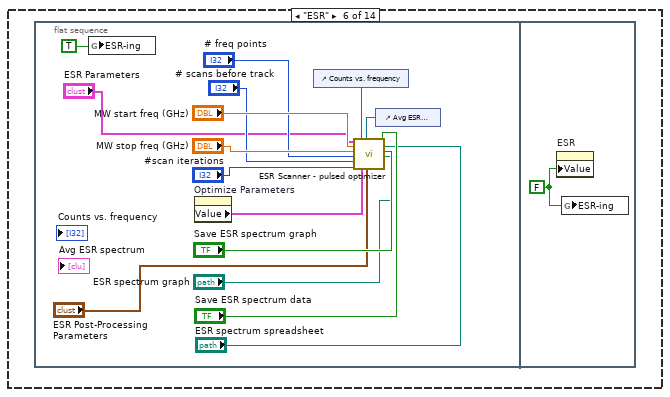
[diagram p12: hidden frame]
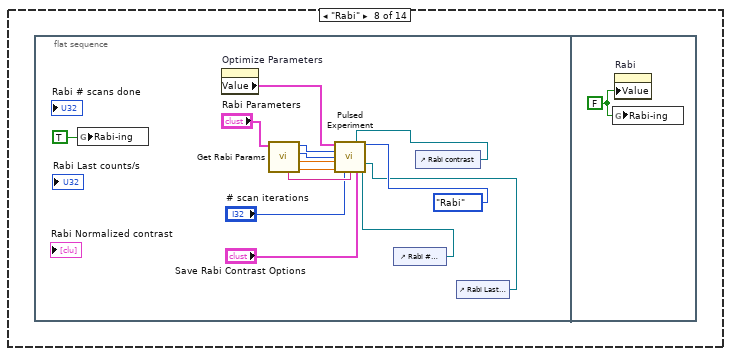
[diagram p13: hidden frame]
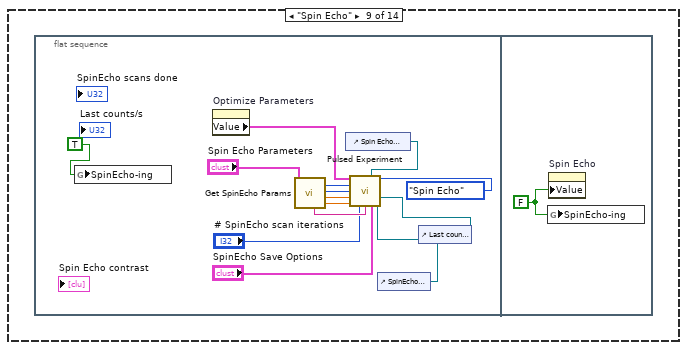
[diagram p14: hidden frame]
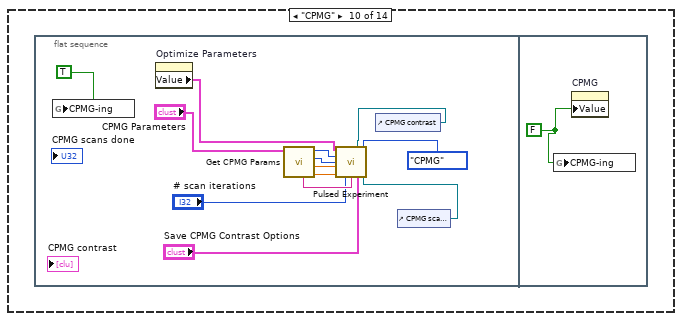
[diagram p15: hidden frame]
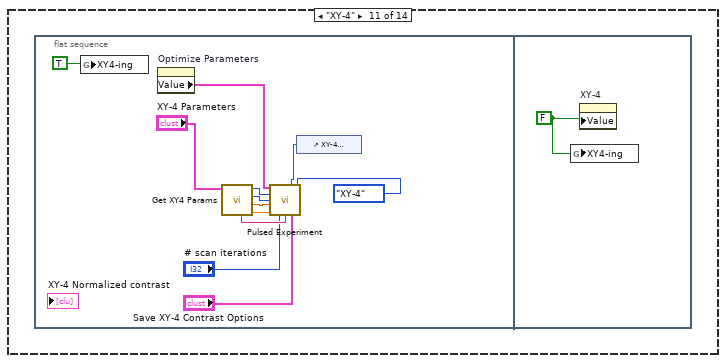
[diagram p16: hidden frame]
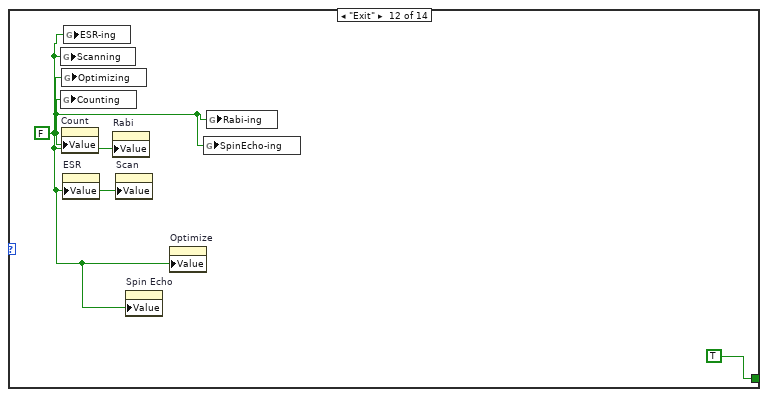
[diagram p17: hidden frame]
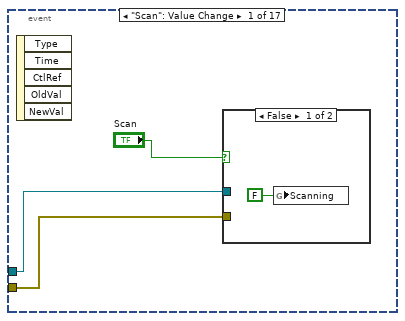
[diagram p20: hidden frame]
diagram:
  w1 = States."Initialize"
  n1 = Obtain Queue(name (unnamed)="Main Queue", element data type=w1) -> (queue out=w4:refnum<queue>, error out=w6:errorcluster)  [unwired: 3 in, 1 out]
  n2 = Enqueue Element(queue=w4, element=w1, error in (no error)=w6) -> (queue out=w3:refnum<queue>, error out=w2:errorcluster)  [unwired: 1 in, 1 out]
  n3 = while {
    tunnel: w3 -> [w9]
    tunnel: w2 -> [w8]
    stop <- w7 stop-if-true
    n4 = Dequeue Element(queue=w9, error in (no error)=w8) -> (element=w10:T14)  [unwired: 1 in, 3 out]
    n5 = case shown="\"ESR 2\"" w10 {
      tunnel: [_ _ _ _ _ _ _ _ _ _ _ TRUE _ _] -> w7
      frame "Initialize" {
        w12 = TRUE
        w11 = FALSE
        n6 = global write "Global Vars.vi" "Scanning"(w11) -> ()
        n7 = global write "Global Vars.vi" "Counting"(w11) -> ()
        n8 = global write "Global Vars.vi" "Optimizing"(w11) -> ()
        n9 = property on="Scan" class="Bool (strict)"("Value"=w11) -> ()  [unwired: 2 in, 2 out]
        n10 = property on="Count" class="Bool (strict)"("Value"=w11) -> ()  [unwired: 2 in, 2 out]
        n11 = global write "Global Vars.vi" "ESR-ing"(w11) -> ()
        n12 = global write "Global Vars.vi" "Rabi-ing"(w11) -> ()
        n13 = property on="Rabi" class="Bool (strict)"("Value"=w11) -> ()  [unwired: 2 in, 2 out]
        n14 = property on="Counts Intensity Graph" class="IntGraph (strict)"("Cursor.Visible"=w12, "YScale.Flipped"=w12) -> ()  [unwired: 2 in, 2 out]
        n15 = property on="ESR" class="Bool (strict)"("Value"=w11) -> ()  [unwired: 2 in, 2 out]
        n16 = property on="Optimize" class="Bool (strict)"("Value"=w11) -> ()  [unwired: 2 in, 2 out]
        n17 = global write "Global Vars.vi" "SpinEcho-ing"(w11) -> ()
        n18 = global write "Global Vars.vi" "Pause SpinEcho"(w11) -> ()
        n19 = property on="CPMG" class="Bool (strict)"("Value"=w11) -> ()  [unwired: 2 in, 2 out]
        n20 = property on="Spin Echo" class="Bool (strict)"("Value"=w11) -> ()  [unwired: 2 in, 2 out]
        n21 = global write "Global Vars.vi" "Pause Rabi"(w11) -> ()
        n22 = global write "Global Vars.vi" "CPMG-ing"(w11) -> ()
        n23 = global write "Global Vars.vi" "XY4-ing"(w11) -> ()
      }
      frame "Scan" {
        n24 = flat-sequence {
          frame #0 {
            w13 = TRUE
            n25 = property on="Counts Intensity Graph" class="IntGraph (strict)"("Cursor.Visible"=FALSE) -> ()  [unwired: 2 in, 2 out]
            n26 = global write "Global Vars.vi" "Scanning"(w13) -> ()
            n27 = property on="Scan" class="Bool (strict)"("Value"=w13) -> ()  [unwired: 2 in, 2 out]
          }
          frame #1 {
            n28 = control-ref of="Counts Intensity Graph"() -> (w23:refnum<vi>)
            n29 = Unbundle By Name("Scan Parameters") -> ("X Max"=w18:dbl, "X Min"=w22:dbl, "X Step"=w21:dbl, "Y Max"=w20:dbl, "Y Min"=w19:dbl, "Y Step"=w16:dbl)
            n30 = property on="Counts Intensity Graph" class="IntGraph (strict)"("XScale.Maximum"=w18, "XScale.Offset"=w22, "XScale.Multiplier"=w21, "YScale.Maximum"=w20, "YScale.Offset"=w19, "YScale.Multiplier"=w16) -> ()  [unwired: 2 in, 2 out]
            n31 = call "Scanner.vi"("Continuous"="Continuous", "IntGraph Refnum"=w23, "Scan Parameters"="Scan Parameters") -> ()  [unwired: 8 in, 1 out]
          }
          frame #2 {
            w24 = FALSE
            n32 = global read "Global Vars.vi" "X Pos"() -> (w26:dbl)
            n33 = global read "Global Vars.vi" "Y Pos"() -> (w25:dbl)
            n34 = call "Update Position to Globals.vi"() -> ()  [unwired: 11 in, 1 out]
            n35 = property on="Counts Intensity Graph" class="IntGraph (strict)"("Cursor.Visible"=TRUE) -> ()  [unwired: 2 in, 2 out]
            n36 = property on="Scan" class="Bool (strict)"("Value"=w24) -> ()  [unwired: 2 in, 2 out]
            n37 = property on="Counts Intensity Graph" class="IntGraph (strict)"("Cursor.Cursor X"=w26, "Cursor.Cursor Y"=w25) -> ()  [unwired: 2 in, 2 out]
            n38 = global write "Global Vars.vi" "Scanning"(w24) -> ()
          }
        }
      }
      frame "Count" {
        n39 = global write "Global Vars.vi" "Counting"(TRUE) -> ()
        n40 = control-ref of="Counts Chart"() -> (w28:refnum<vi>)
        n41 = control-ref of="Counts/s"() -> (w29:refnum<vi>)
        n42 = call "Counter.vi"("Counts Chart Refnum"=w28, "Counts/s Ref"=w29) -> ()  [unwired: 10 in]
      }
      frame "Optimize" {
        n43 = flat-sequence {
          frame #0 {
            w32 = TRUE
            n44 = property on="Count" class="Bool (strict)"() -> ("Value"=w31:bool)  [unwired: 2 in, 2 out]
            n45 = case shown="True" w31 {
              frame False {
              }
              frame True {
                n46 = global write "Global Vars.vi" "Counting"(TRUE) -> ()
              }
            }
            n47 = global write "Global Vars.vi" "Optimizing"(w32) -> ()
            n48 = property on="Optimize" class="Bool (strict)"("Value"=w32) -> ()  [unwired: 2 in, 2 out]
          }
          frame #1 {
            n49 = flat-sequence {
              frame #0 {
                n50 = call "Optimizer.vi"("Optimize Parameters"="Optimize Parameters") -> ()  [unwired: 10 in, 1 out]
              }
              frame #1 {
                w41 = FALSE
                n51 = global read "Global Vars.vi" "X Pos"() -> (w44:dbl)
                n52 = global read "Global Vars.vi" "Y Pos"() -> (w43:dbl)
                n53 = property on="Counts Intensity Graph" class="IntGraph (strict)"("Cursor.Cursor X"=w44, "Cursor.Cursor Y"=w43) -> ()  [unwired: 2 in, 2 out]
                n54 = global read "Global Vars.vi" "Z Pos"() -> (w42:dbl)
                n55 = property on="Z Voltage" class="DigNum (strict)"("Value"=w42) -> ()  [unwired: 2 in, 2 out]
                n56 = property on="Optimize" class="Bool (strict)"("Value"=w41) -> ()  [unwired: 2 in, 2 out]
                n57 = global write "Global Vars.vi" "Optimizing"(w41) -> ()
              }
            }
            n58 = while {
              stop <- w39 stop-if-true
              n59 = global read "Global Vars.vi" "X Pos"() -> (w37:dbl)
              n60 = global read "Global Vars.vi" "Y Pos"() -> (w36:dbl)
              n61 = global read "Global Vars.vi" "Z Pos"() -> (w34:dbl)
              n62 = global read "Global Vars.vi" "Optimizing"() -> (w38:bool)
              n63 = property on="Counts Intensity Graph" class="IntGraph (strict)"("Cursor.Cursor X"=w37, "Cursor.Cursor Y"=w36) -> ()  [unwired: 2 in, 2 out]
              n64 = property on="Z Voltage" class="DigNum (strict)"("Value"=w34) -> ()  [unwired: 2 in, 2 out]
              n65 = Not(x=w38) -> (.not. x?=w39:bool)
              n66 = Wait (ms)(milliseconds to wait=u32 100 ("millisecond multiple")) -> ()  [unwired: 1 out]
            }
          }
        }
      }
      frame "Hold" {
        # "Boolean array for\nchannel outputs"
        n67 = global read "Channels.vi" "spinapi.dll"() -> (w51:path)
        n68 = Build Array("Microwave", "Green Laser (low-T)", FALSE, "Green Laser") -> (w45:bool[])
        n69 = Or Array Elements(Boolean array=w45) -> (logical OR=w50:bool)
        n70 = case shown="True" w50 {
          tunnel: w51 -> [w52 w54]
          tunnel: w45 -> [_ w53]
          frame False {
            n71 = call "PB_reset.vi"("Path to spinapi.dll"=w52) -> ()  [unwired: 7 in]
          }
          frame True {
            n72 = flat-sequence {
              tunnel: w53 -> [w55]
              tunnel: w54 -> [w56]
              frame #0 {
                n73 = call "PB_Cburn_hold.vi"("Optimize active channels"=w55) -> ()  [unwired: 9 in, 2 out]
              }
              frame #1 {
                n74 = call "PB_blast.vi"("Path to spinapi.dll"=w56) -> ()  [unwired: 7 in]
              }
            }
          }
        }
      }
      frame "ESR" {
        n75 = flat-sequence {
          frame #0 {
            n76 = global write "Global Vars.vi" "ESR-ing"(TRUE) -> ()
            n77 = property on="Optimize Parameters" class="Clust (strict)"() -> ("Value"=w62:T3)  [unwired: 2 in, 2 out]
            n78 = control-ref of="Counts vs. frequency"() -> (w64:refnum<vi>)
            n79 = control-ref of="Avg ESR spectrum"() -> (w63:refnum<vi>)
            n80 = call "ESR Scanner - pulsed optimizer.vi"("ESR Parameters"="ESR Parameters", "MW start freq (GHz)"="MW start freq (GHz)", "MW stop freq (GHz)"="MW stop freq (GHz)", "# freq points"="# freq points", "# scans before track"="# scans before track", "#scan iterations"="#scan iterations", "IntGraph Refnum"=w64, "Optimize Parameters"=w62, "XY Graph Refnum"=w63, "ESR Post-Processing Parameters"="ESR Post-Processing Parameters", "Save avg spectrum data to spreadsheet?"="Save ESR spectrum data", "Path for avg spectrum spreadsheet"="ESR spectrum spreadsheet", "Save avg spectrum graph?"="Save ESR spectrum graph", "Path for avg spectrum graph"="ESR spectrum graph") -> ()  [unwired: 6 in]
          }
          frame #1 {
            w72 = FALSE
            n81 = property on="ESR" class="Bool (strict)"("Value"=w72) -> ()  [unwired: 2 in, 2 out]
            n82 = global write "Global Vars.vi" "ESR-ing"(w72) -> ()
          }
        }
      }
      frame "ESR 2" {
        n83 = flat-sequence {
          frame #0 {
            n84 = property on="Optimize Parameters" class="Clust (strict)"() -> ("Value"=w80:T3)  [unwired: 2 in, 2 out]
            n85 = global write "Global Vars.vi" "ESR 2-ing"(TRUE) -> ()
            n86 = control-ref of="Counts vs. frequency 2-1"() -> (w76:refnum<vi>)
            n87 = control-ref of="Avg ESR spectrum 2-1"() -> (w75:refnum<vi>)
            n88 = control-ref of="Counts vs. frequency 2-2"() -> (w74:refnum<vi>)
            n89 = control-ref of="Avg ESR spectrum 2-2"() -> (w73:refnum<vi>)
            n90 = call "ESR Scanner - modified.vi"("ESR Modified Parameters"="ESR Modified Parameters", "MW start freq (GHz)"="MW start freq (GHz) 2", "MW stop freq (GHz)"="MW stop freq (GHz) 2", "# freq points"="# freq points 2", "# scans before track"="# scans before track 2", "#scan iterations"="#scan iterations 2", "IntGraph Refnum"=w76, "Optimize Parameters"=w80, "XY Graph Refnum"=w75, "ESR Post-Processing Parameters"="ESR Post-Processing Parameters 2", "IntGraph Refnum 2"=w74, "Data 1"="ESR Save Data 1", "XY Graph Refnum 2"=w73, "Data 2"="ESR Save Data 2") -> ()  [unwired: 6 in]
          }
          frame #1 {
            w88 = FALSE
            n91 = property on="ESR 2" class="Bool (strict)"("Value"=w88) -> ()  [unwired: 2 in, 2 out]
            n92 = global write "Global Vars.vi" "ESR 2-ing"(w88) -> ()
          }
        }
      }
      frame "Rabi" {
        n93 = flat-sequence {
          frame #0 {
            n94 = global write "Global Vars.vi" "Rabi-ing"(TRUE) -> ()
            n95 = property on="Optimize Parameters" class="Clust (strict)"() -> ("Value"=w95:T3)  [unwired: 2 in, 2 out]
            n96 = call "Get Rabi Params.vi"("Rabi Parameters"="Rabi Parameters") -> ("max time"=w98:dbl, "min time"=w99:dbl, "# time points"=w100:i32, "# samples"=w101:i32, "PB Window Args"=w97:string)  [unwired: 6 in]
            n97 = control-ref of="Rabi # scans done"() -> (w90:refnum<vi>)
            n98 = control-ref of="Rabi contrast"() -> (w92:refnum<vi>)
            n99 = control-ref of="Rabi Last counts/s"() -> (w89:refnum<vi>)
            n100 = call "Pulsed Experiment.vi"("Optimize Parameters"=w95, "Contrast XY Graph Refnum"=w92, "Experiment"=States."Rabi", "# samples"=w101, "# time points"=w100, "min time"=w99, "Last counts/s ref"=w89, "max time"=w98, "# scan iterations"="# scan iterations", "Window Parameters"=w97, "Save Contrast Options"="Save Rabi Contrast Options", "scans done ref"=w90) -> ()  [unwired: 4 in]
          }
          frame #1 {
            w103 = FALSE
            n101 = global write "Global Vars.vi" "Rabi-ing"(w103) -> ()
            n102 = property on="Rabi" class="Bool (strict)"("Value"=w103) -> ()  [unwired: 2 in, 2 out]
          }
        }
      }
      frame "Spin Echo" {
        n103 = flat-sequence {
          frame #0 {
            n104 = global write "Global Vars.vi" "SpinEcho-ing"(TRUE) -> ()
            n105 = property on="Optimize Parameters" class="Clust (strict)"() -> ("Value"=w115:T3)  [unwired: 2 in, 2 out]
            n106 = call "Get SpinEcho Params.vi"("Spin Echo Parameters"="Spin Echo Parameters") -> ("max time"=w111:dbl, "min time"=w112:dbl, "# time points"=w113:i32, "# samples"=w114:i32, "Window Params Args"=w110:string)  [unwired: 6 in]
            n107 = control-ref of="Spin Echo contrast"() -> (w107:refnum<vi>)
            n108 = control-ref of="SpinEcho scans done"() -> (w105:refnum<vi>)
            n109 = control-ref of="Last counts/s"() -> (w104:refnum<vi>)
            n110 = call "Pulsed Experiment.vi"("Optimize Parameters"=w115, "Contrast XY Graph Refnum"=w107, "Experiment"=States."Spin Echo", "# samples"=w114, "# time points"=w113, "min time"=w112, "Last counts/s ref"=w104, "max time"=w111, "# scan iterations"="# SpinEcho scan iterations", "Window Parameters"=w110, "Save Contrast Options"="SpinEcho Save Options", "scans done ref"=w105) -> ()  [unwired: 4 in]
          }
          frame #1 {
            w118 = FALSE
            n111 = global write "Global Vars.vi" "SpinEcho-ing"(w118) -> ()
            n112 = property on="Spin Echo" class="Bool (strict)"("Value"=w118) -> ()  [unwired: 2 in, 2 out]
          }
        }
      }
      frame "CPMG" {
        n113 = flat-sequence {
          frame #0 {
            n114 = global write "Global Vars.vi" "CPMG-ing"(TRUE) -> ()
            n115 = property on="Optimize Parameters" class="Clust (strict)"() -> ("Value"=w119:T3)  [unwired: 2 in, 2 out]
            n116 = call "Get CPMG Params.vi"("CPMG Parameters"="CPMG Parameters") -> ("max time"=w130:dbl, "min time"=w129:dbl, "# time points"=w128:i32, "# samples"=w127:i32, "Window Params Args"=w126:string)  [unwired: 6 in]
            n117 = control-ref of="CPMG contrast"() -> (w122:refnum<vi>)
            n118 = control-ref of="CPMG scans done"() -> (w120:refnum<vi>)
            n119 = call "Pulsed Experiment.vi"("Optimize Parameters"=w119, "Contrast XY Graph Refnum"=w122, "Experiment"=States."CPMG", "# samples"=w127, "# time points"=w128, "min time"=w129, "max time"=w130, "# scan iterations"="# scan iterations", "Window Parameters"=w126, "Save Contrast Options"="Save CPMG Contrast Options", "scans done ref"=w120) -> ()  [unwired: 5 in]
          }
          frame #1 {
            w132 = FALSE
            n120 = global write "Global Vars.vi" "CPMG-ing"(w132) -> ()
            n121 = property on="CPMG" class="Bool (strict)"("Value"=w132) -> ()  [unwired: 2 in, 2 out]
          }
        }
      }
      frame "XY-4" {
        n122 = flat-sequence {
          frame #0 {
            n123 = global write "Global Vars.vi" "XY4-ing"(TRUE) -> ()
            n124 = property on="Optimize Parameters" class="Clust (strict)"() -> ("Value"=w138:T3)  [unwired: 2 in, 2 out]
            n125 = call "Get XY4 Params.vi"("XY-4 Parameters"="XY-4 Parameters") -> ("max time"=w140:dbl, "min time"=w141:dbl, "# time points"=w142:i32, "# samples"=w143:i32, "String"=w139:string)  [unwired: 6 in]
            n126 = control-ref of="XY-4 Normalized contrast"() -> (w134:refnum<vi>)
            n127 = call "Pulsed Experiment.vi"("Optimize Parameters"=w138, "Contrast XY Graph Refnum"=w134, "Experiment"=States."XY-4", "# samples"=w143, "# time points"=w142, "min time"=w141, "max time"=w140, "# scan iterations"="# scan iterations", "Window Parameters"=w139, "Save Contrast Options"="Save XY-4 Contrast Options") -> ()  [unwired: 6 in]
          }
          frame #1 {
            w145 = FALSE
            n128 = global write "Global Vars.vi" "XY4-ing"(w145) -> ()
            n129 = property on="XY-4" class="Bool (strict)"("Value"=w145) -> ()  [unwired: 2 in, 2 out]
          }
        }
      }
      frame "Exit" {
        w146 = FALSE
        n130 = global write "Global Vars.vi" "Scanning"(w146) -> ()
        n131 = global write "Global Vars.vi" "Counting"(w146) -> ()
        n132 = global write "Global Vars.vi" "Optimizing"(w146) -> ()
        n133 = property on="Count" class="Bool (strict)"("Value"=w146) -> ()  [unwired: 2 in, 2 out]
        n134 = property on="ESR" class="Bool (strict)"("Value"=w146) -> ()  [unwired: 2 in, 2 out]
        n135 = global write "Global Vars.vi" "ESR-ing"(w146) -> ()
        n136 = property on="Rabi" class="Bool (strict)"("Value"=w146) -> ()  [unwired: 2 in, 2 out]
        n137 = property on="Scan" class="Bool (strict)"("Value"=w146) -> ()  [unwired: 2 in, 2 out]
        n138 = property on="Spin Echo" class="Bool (strict)"("Value"=w146) -> ()  [unwired: 2 in, 2 out]
        n139 = property on="Optimize" class="Bool (strict)"("Value"=w146) -> ()  [unwired: 2 in, 2 out]
        n140 = global write "Global Vars.vi" "SpinEcho-ing"(w146) -> ()
        n141 = global write "Global Vars.vi" "Rabi-ing"(w146) -> ()
      }
      frame "Spectrum" {
      }
      frame "Stability" {
      }
    }
  }
  n142 = while {
    tunnel: w3 -> [w150]
    tunnel: w2 -> [w149]
    stop <- w148 stop-if-true
    n143 = event shown="[6] \"ESR 2\": Value Change" {
      selector: _ -> [_ _ _ _ _ _ _ _ _ _ _ _ _ _ _ _ _]
      dyn-events: _ -> [_ _ _ _ _ _ _ _ _ _ _ _ _ _ _ _ _]
      timeout: _ -> [_ _ _ _ _ _ _ _ _ _ _ _ _ _ _ _ _]
      tunnel: w150 -> [w152 w159 w167 _ _ w185 w193 w201 _ _ w212 w216 _ _ w233 w240 w248]
      tunnel: w149 -> [w151 w158 w166 _ _ w186 w192 w200 _ _ w211 w215 _ _ w234 w239 w247]
      tunnel: [_ _ _ _ _ _ _ _ _ _ TRUE _ _ _ _ _ _] -> w148
      event "Scan": Value Change {
        n144 = event-data() -> ()  [unwired: 1 in, 5 out]
        n145 = case shown="False" "Scan" {
          tunnel: w152 -> [_ w156]
          tunnel: w151 -> [_ w155]
          frame False {
            n146 = global write "Global Vars.vi" "Scanning"(FALSE) -> ()
          }
          frame True {
            n147 = Enqueue Element(queue=w156, element=States."Scan", error in (no error)=w155) -> ()  [unwired: 1 in, 3 out]
          }
        }
      }
      event "Optimize": Value Change {
        n148 = event-data() -> ()  [unwired: 1 in, 5 out]
        n149 = case shown="True" "Optimize" {
          tunnel: w159 -> [_ w163]
          tunnel: w158 -> [_ w162]
          frame False {
          }
          frame True {
            n150 = global write "Global Vars.vi" "Counting"(FALSE) -> ()
            n151 = Enqueue Element(queue=w163, element=States."Optimize", error in (no error)=w162) -> ()  [unwired: 1 in, 3 out]
          }
        }
      }
      event "Count": Value Change {
        n152 = event-data() -> ()  [unwired: 1 in, 5 out]
        n153 = case shown="True" "Count" {
          tunnel: w167 -> [_ w170]
          tunnel: w166 -> [_ w169]
          frame False {
            n154 = global write "Global Vars.vi" "Counting"(FALSE) -> ()
          }
          frame True {
            n155 = global read "Global Vars.vi" "Pause SpinEcho"() -> (w174:bool)
            n156 = global read "Global Vars.vi" "Optimizing"() -> (w173:bool)
            n157 = global read "Global Vars.vi" "Pause Rabi"() -> (w175:bool)
            n158 = Or(x=w175, y=w174) -> (x .or. y?=w172:bool)
            n159 = Or(x=w173, y=w172) -> (x .or. y?=w171:bool)
            n160 = case shown="False" w171 {
              tunnel: w170 -> [w177 _]
              tunnel: w169 -> [w176 _]
              frame False {
                n161 = Enqueue Element(queue=w177, element=States."Count", error in (no error)=w176) -> ()  [unwired: 1 in, 3 out]
              }
              frame True {
                n162 = global write "Global Vars.vi" "Counting"(TRUE) -> ()
              }
            }
          }
        }
      }
      event "Counts Intensity Graph": Cursor Release; "Counts Intensity Graph": Cursor Move {
        n163 = event-data() -> ("CursLoc"=w180:cluster{"X":dbl, "Y":dbl})  [unwired: 1 in, 7 out]
        n164 = flat-sequence {
          tunnel: w180 -> [w181]
          frame #0 {
            n165 = Unbundle By Name(w181) -> ("X"=w183:dbl, "Y"=w182:dbl)
            n166 = global write "Global Vars.vi" "X Pos"(w183) -> ()
            n167 = global write "Global Vars.vi" "Y Pos"(w182) -> ()
          }
          frame #1 {
            n168 = call "Update Position to Globals.vi"() -> ()  [unwired: 11 in, 1 out]
          }
        }
      }
      event "Z Voltage": Value Change {
        n169 = event-data() -> ()  [unwired: 1 in, 5 out]
        n170 = flat-sequence {
          frame #0 {
            n171 = global write "Global Vars.vi" "Z Pos"("Z Voltage") -> ()
          }
          frame #1 {
            n172 = call "Update Position to Globals.vi"() -> ()  [unwired: 11 in, 1 out]
          }
        }
      }
      event "ESR": Value Change {
        n173 = event-data() -> ()  [unwired: 1 in, 5 out]
        n174 = case shown="True" "ESR" {
          tunnel: w185 -> [_ w190]
          tunnel: w186 -> [_ w189]
          frame False {
            n175 = global write "Global Vars.vi" "ESR-ing"(FALSE) -> ()
          }
          frame True {
            n176 = Enqueue Element(queue=w190, element=States."ESR", error in (no error)=w189) -> ()  [unwired: 1 in, 3 out]
          }
        }
      }
      event "ESR 2": Value Change {
        n177 = event-data() -> ()  [unwired: 1 in, 5 out]
        n178 = case shown="False" "ESR 2" {
          tunnel: w193 -> [_ w197]
          tunnel: w192 -> [_ w196]
          frame False {
            n179 = global write "Global Vars.vi" "ESR 2-ing"(FALSE) -> ()
          }
          frame True {
            n180 = Enqueue Element(queue=w197, element=States."ESR 2", error in (no error)=w196) -> ()  [unwired: 1 in, 3 out]
          }
        }
      }
      event "Green Laser", "Microwave", "Green Laser (low-T)": Value Change {
        n181 = event-data() -> ()  [unwired: 1 in, 5 out]
        n182 = Enqueue Element(queue=w201, element=States."Hold", error in (no error)=w200) -> ()  [unwired: 1 in, 3 out]
      }
      event Timeout {
        n183 = event-data() -> ()  [unwired: 1 in, 2 out]
      }
      event "Z AO Channel", "Y AO Channel", "Counter(s)", "Sample clock line", "spinapi.dll", "HoldChannel.exe", "Laser voltage", "X AO Channel": Value Change {
        n184 = event-data() -> ()  [unwired: 1 in, 5 out]
        n185 = global write "Channels.vi" "Laser voltage"("Laser voltage") -> ()
        n186 = global write "Channels.vi" "X Channel"("X AO Channel") -> ()
        n187 = global write "Channels.vi" "Y Channel"("Y AO Channel") -> ()
        n188 = global write "Channels.vi" "Counter(s)"("Counter(s)") -> ()
        n189 = global write "Channels.vi" "Sample clock line"("Sample clock line") -> ()
        n190 = global write "Channels.vi" "HoldChannel.exe"("HoldChannel.exe") -> ()
        n191 = global write "Channels.vi" "spinapi.dll"("spinapi.dll") -> ()
        n192 = global write "Channels.vi" "Z Channel"("Z AO Channel") -> ()
      }
      event Panel Close? {
        w210 = FALSE
        n193 = event-data() -> ()  [unwired: 1 in, 3 out]
        n194 = Enqueue Element(queue=w212, element=States."Exit", error in (no error)=w211) -> ()  [unwired: 1 in, 3 out]
        n195 = global write "Global Vars.vi" "Optimizing"(w210) -> ()
        n196 = global write "Global Vars.vi" "Scanning"(w210) -> ()
        n197 = global write "Global Vars.vi" "Counting"(w210) -> ()
        n198 = global write "Global Vars.vi" "ESR-ing"(w210) -> ()
        n199 = event-data() -> ()  [unwired: 2 in, 1 out]
      }
      event "Rabi": Value Change {
        n200 = event-data() -> ()  [unwired: 1 in, 5 out]
        n201 = case shown="False" "Rabi" {
          tunnel: w216 -> [_ w220]
          tunnel: w215 -> [_ w219]
          frame False {
            n202 = global write "Global Vars.vi" "Rabi-ing"(FALSE) -> ()
          }
          frame True {
            n203 = Enqueue Element(queue=w220, element=States."Rabi", error in (no error)=w219) -> ()  [unwired: 1 in, 3 out]
          }
        }
      }
      event "Rabi Pause": Value Change {
        n204 = event-data() -> ()  [unwired: 1 in, 5 out]
        n205 = case shown="False" "Rabi Pause" {
          frame False {
            n206 = while {
              stop <- w224 continue-if-true
              n207 = property on="Count" class="Bool (strict)"() -> ("Value"=w224:bool)  [unwired: 2 in, 2 out]
              n208 = case shown="False" w224 {
                frame False {
                  n209 = global write "Global Vars.vi" "Pause Rabi"(FALSE) -> ()
                }
                frame True {
                }
              }
            }
            n210 = global write "Global Vars.vi" "Counting"(FALSE) -> ()
          }
          frame True {
            n211 = global write "Global Vars.vi" "Pause Rabi"(TRUE) -> ()
          }
        }
      }
      event "Pause Spin Echo": Value Change {
        n212 = event-data() -> ()  [unwired: 1 in, 5 out]
        n213 = case shown="False" "Pause Spin Echo" {
          frame False {
            n214 = while {
              stop <- w229 continue-if-true
              n215 = property on="Count" class="Bool (strict)"() -> ("Value"=w229:bool)  [unwired: 2 in, 2 out]
              n216 = case shown="False" w229 {
                frame False {
                  n217 = global write "Global Vars.vi" "Pause SpinEcho"(FALSE) -> ()
                }
                frame True {
                }
              }
            }
            n218 = global write "Global Vars.vi" "Counting"(FALSE) -> ()
          }
          frame True {
            n219 = global write "Global Vars.vi" "Pause SpinEcho"(TRUE) -> ()
          }
        }
      }
      event "Spin Echo": Value Change {
        n220 = event-data() -> ()  [unwired: 1 in, 5 out]
        n221 = case shown="True" "Spin Echo" {
          tunnel: w233 -> [_ w237]
          tunnel: w234 -> [_ w236]
          frame False {
            n222 = global write "Global Vars.vi" "SpinEcho-ing"(FALSE) -> ()
          }
          frame True {
            n223 = Enqueue Element(queue=w237, element=States."Spin Echo", error in (no error)=w236) -> ()  [unwired: 1 in, 3 out]
          }
        }
      }
      event "CPMG": Value Change {
        n224 = event-data() -> ()  [unwired: 1 in, 5 out]
        n225 = case shown="True" "CPMG" {
          tunnel: w240 -> [_ w244]
          tunnel: w239 -> [_ w243]
          frame False {
            n226 = global write "Global Vars.vi" "CPMG-ing"(FALSE) -> ()
          }
          frame True {
            n227 = Enqueue Element(queue=w244, element=States."CPMG", error in (no error)=w243) -> ()  [unwired: 1 in, 3 out]
          }
        }
      }
      event "XY-4": Value Change {
        n228 = event-data() -> ()  [unwired: 1 in, 5 out]
        n229 = case shown="True" "XY-4" {
          tunnel: w248 -> [_ w251]
          tunnel: w247 -> [_ w250]
          frame False {
            n230 = global write "Global Vars.vi" "XY4-ing"(FALSE) -> ()
          }
          frame True {
            n231 = Enqueue Element(queue=w251, element=States."XY-4", error in (no error)=w250) -> ()  [unwired: 1 in, 3 out]
          }
        }
      }
    }
  }
  n232 = while {
    stop <- FALSE stop-if-true
    n233 = global read "Global Vars.vi" "Counting"() -> (w254:bool)
    n234 = case shown="True" w254 {
      frame False {
      }
      frame True {
        n235 = global read "Global Vars.vi" "Optimizing"() -> (w256:bool)
        n236 = case shown="True" w256 {
          frame False {
            n237 = global read "Global Vars.vi" "Pause SpinEcho"() -> (w258:bool)
            n238 = global read "Global Vars.vi" "Pause Rabi"() -> (w259:bool)
            n239 = Or(x=w259, y=w258) -> (x .or. y?=w257:bool)
            n240 = case shown="True" w257 {
              frame False {
              }
              frame True {
                n241 = flat-sequence {
                  frame #0 {
                    n242 = control-ref of="Counts Chart"() -> (w260:refnum<vi>)
                    n243 = control-ref of="Counts/s"() -> (w261:refnum<vi>)
                    n244 = call "Counter.vi"("Counts Chart Refnum"=w260, "Counts/s Ref"=w261) -> ()  [unwired: 10 in]
                  }
                  frame #1 {
                    n245 = property on="Count" class="Bool (strict)"("Value"=FALSE) -> ()  [unwired: 2 in, 2 out]
                  }
                }
              }
            }
          }
          frame True {
            n246 = while {
              stop <- w263 stop-if-true
              n247 = global read "Global Vars.vi" "Counts"() -> (w266:u32)
              n248 = global read "Global Vars.vi" "Optimizing"() -> (w265:bool)
              n249 = property on="Counts Chart" class="WFChart (strict)"("Value"=w266) -> ()  [unwired: 2 in, 2 out]
              n250 = property on="Counts/s" class="DigNum (strict)"("Value"=w266) -> ()  [unwired: 2 in, 2 out]
              n251 = global read "Global Vars.vi" "Counting"() -> (w264:bool)
              n252 = Not And(1:w264, 2:w265) -> (0:w263:bool)
              n253 = Wait (ms)(milliseconds to wait=100) -> ()  [unwired: 1 out]
            }
          }
        }
      }
    }
    n254 = Wait (ms)(milliseconds to wait=10) -> ()  [unwired: 1 out]
  }
